vi "Write Device Functional.vi"(8 "error in (no error)":errorcluster, 10 "Device Functional":bool, 11 "DAQdevice in":refnum<class "DAQdevice.lvclass">) -> (0 "error out":errorcluster, 3 "DAQdevice out":refnum<class "DAQdevice.lvclass">)   [LabVIEW 2016, in "DAQdevice.lvclass"]
uses:
  DAQdevice.lvclass
  DAQdevice.lvclass/DAQdevice.ctl
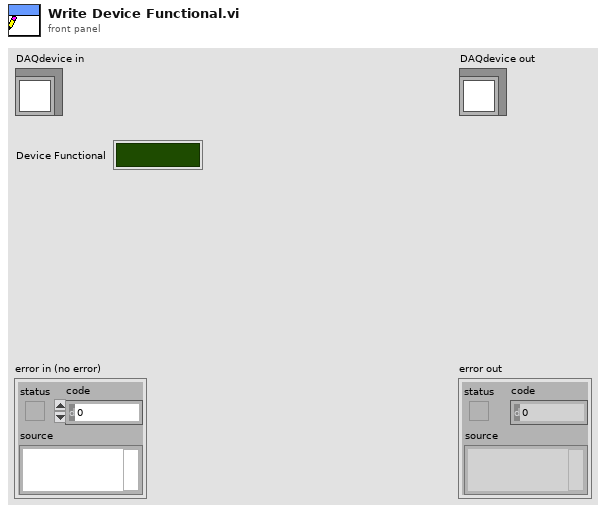
[diagram p1: front panel]
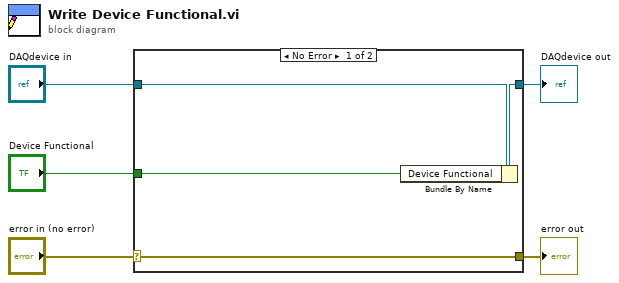
[diagram p0: block diagram]
diagram:
  n1 = case shown="No Error" "error in (no error)" {
    selector: "error in (no error)" -> [w9 w10]
    tunnel: [w9 w10] -> w4
    tunnel: [w7 w11] -> w2
    tunnel: "DAQdevice in" -> [w8 w11]
    tunnel: "Device Functional" -> [w6 _]
    frame No Error {
      n2 = Bundle By Name(cluster=w8, "Device Functional"=w6) -> (w7:refnum<class "DAQdevice.lvclass">)
    }
    frame Error {
    }
  }
  "error out" <- w4
  "DAQdevice out" <- w2
